vi "CreateTriggerNode.vi"(7 "DOM Document":refnum<k20>, 8 "Error In":errorcluster, 11 "Trigger Configuration":T1={"Input"={"Type"=enum."None", "Timeout (ms)"=1, "Delay (ms)"=0, "Digital IO Line (1-14)"=0, "Digital IO Mode"=enum."Falling"}, "Output"={"Type"=enum."None", "Delay (ms)"=0, "Digital IO Line (1-14)"=1, "Digital IO Mode"=enum."Falling", "Digital IO Pulse Width (sec)"=0.0}} {"Output"."Digital IO Line (1-14)" min=1 max=14 step=1}) -> (0 "Error Out":errorcluster, 3 "Trigger Node":refnum<k20>)   [LabVIEW 2012]
uses:
  TriggerConfiguration.ctl
  TriggerInputConfiguration.ctl
  TriggerInputType.ctl
  driver/Public/Controls/TriggerMode.ctl
  TriggerOutputConfiguration.ctl
  TriggerOutputType.ctl
  libs/LV-Utilities/LV-Utilities.lvlib
  driver/Keithley-2602.lvlib
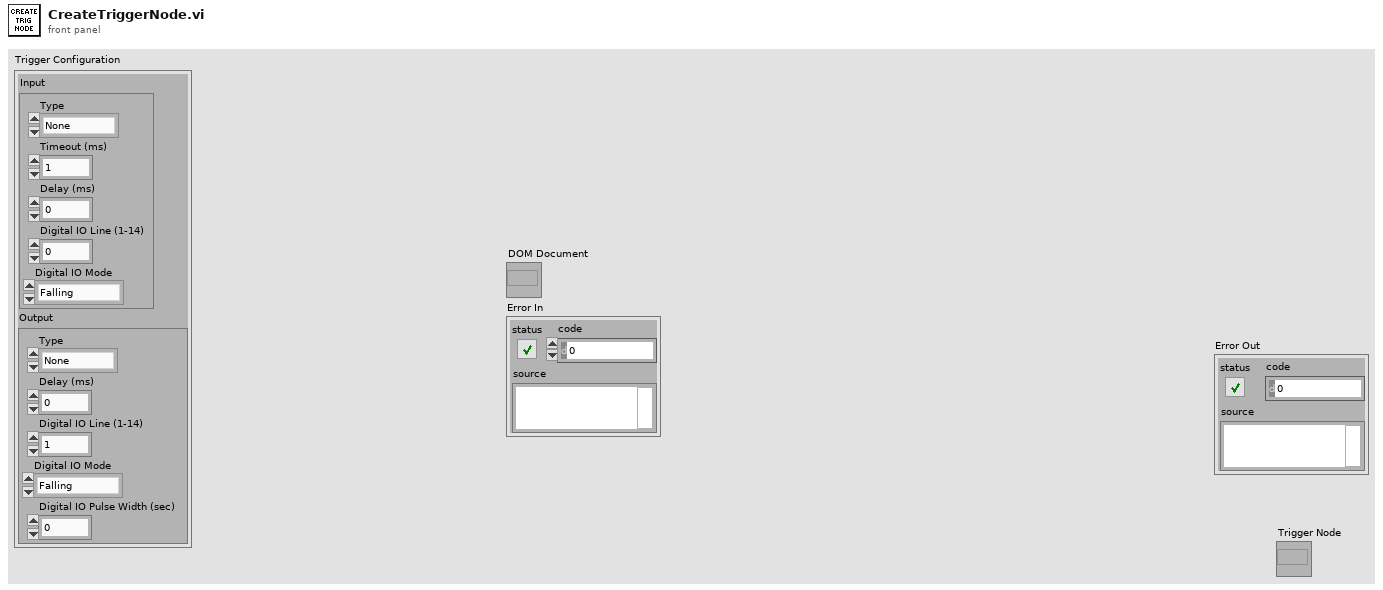
[diagram p1: front panel]
types:
  T1 = typedef "TriggerConfiguration.ctl" = cluster{"Input":T2, "Output":T5}
  T2 = typedef "TriggerInputConfiguration.ctl" = cluster{"Type":T3, "Timeout (ms)":u32, "Delay (ms)":u32, "Digital IO Line (1-14)":u8, "Digital IO Mode":T4}
  T3 = typedef "TriggerInputType.ctl" = enum16{"None", "Digital IO", "Bus"}
  T4 = typedef "Keithley-2602.lvlib/TriggerMode.ctl" = enum16{"Falling", "Rising", "Either", "Synchronous"}
  T5 = typedef "TriggerOutputConfiguration.ctl" = cluster{"Type":T6, "Delay (ms)":u32, "Digital IO Line (1-14)":u8, "Digital IO Mode":T4, "Digital IO Pulse Width (sec)":dbl}
  T6 = typedef "TriggerOutputType.ctl" = enum16{"None", "Digital IO", "Bus"}
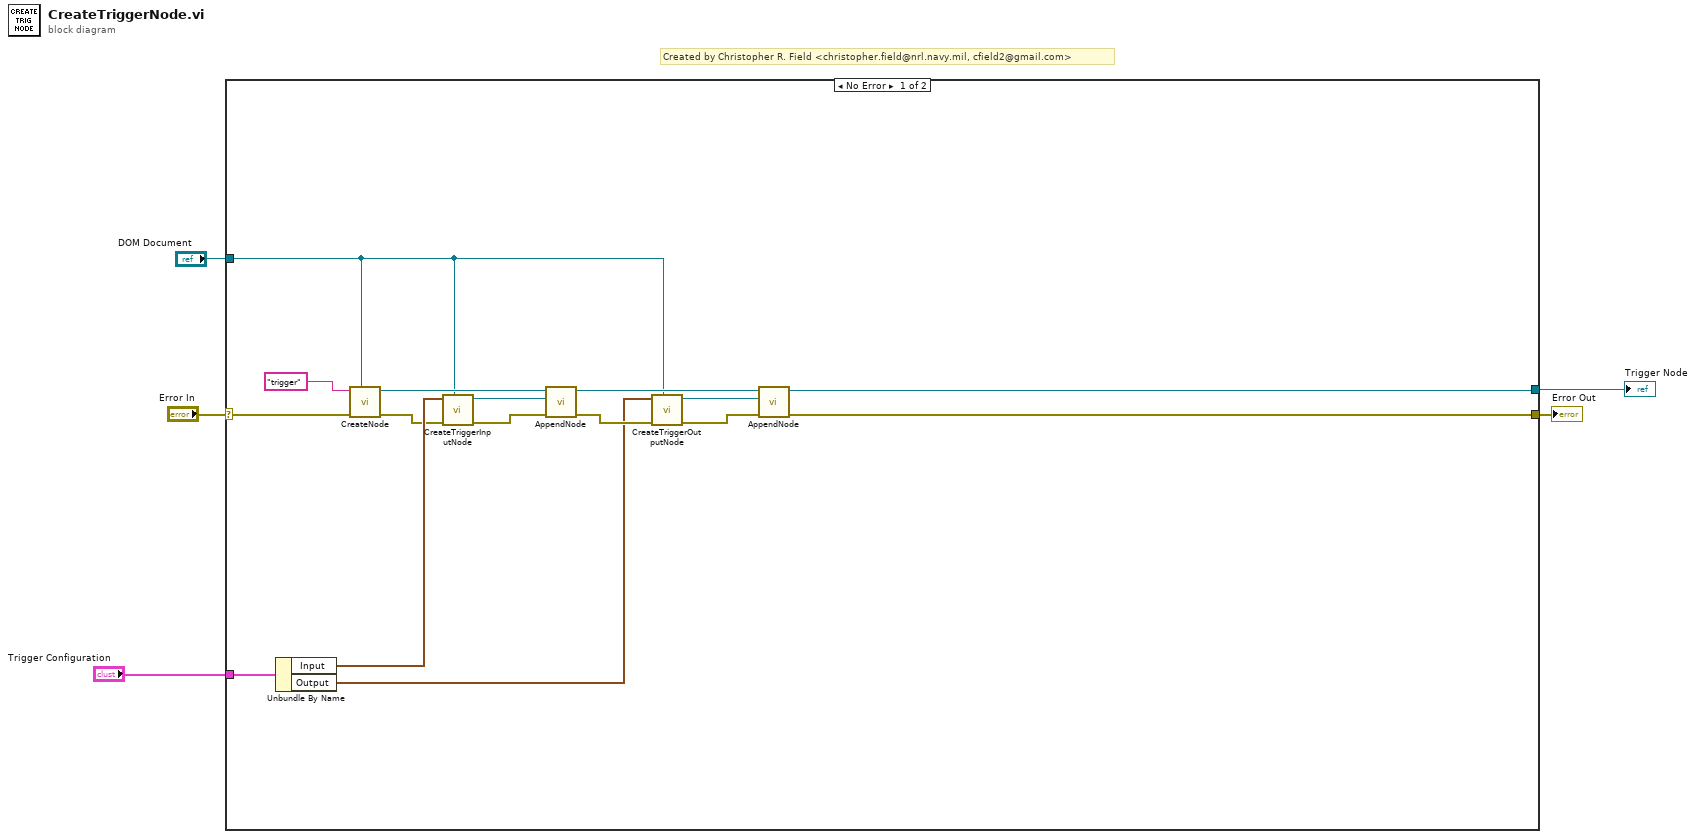
[diagram p0: block diagram]
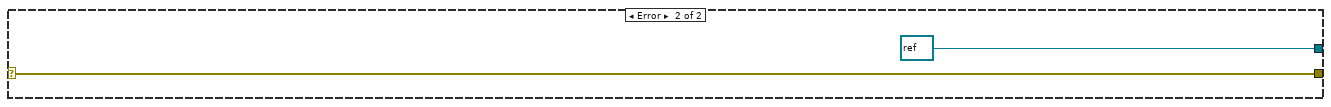
[diagram p2: hidden frame]
diagram:
  # "Created by Christopher R. Field <christopher.field@nrl.navy.mil, cfield2@gmail.com>"
  n1 = case shown="No Error" "Error In" {
    selector: "Error In" -> [w21 w23]
    tunnel: "DOM Document" -> [w9 _]
    tunnel: [w11 w23] -> w3
    tunnel: [w12 refnum<k20> refnum ("DUT Node 2")] -> w2
    tunnel: "Trigger Configuration" -> [w17 _]
    frame No Error {
      n2 = Unbundle By Name(w17) -> ("Input"=w16:T2, "Output"=w8:T5)
      n3 = call "CreateNode.vi"("DOM Document"=w9, "Error In"=w21, "Tag Name"="trigger") -> ("Error out"=w15:errorcluster, "Node"=w19:refnum<k20>)  [unwired: 7 in]
      n4 = call "CreateTriggerInputNode.vi"("DOM Document"=w9, "Error In"=w15, "Trigger Input Configuration"=w16) -> ("Error Out"=w13:errorcluster, "Trigger Input Node"=w14:refnum<k20>)  [unwired: 7 in]
      n5 = call "AppendNode.vi"("Error In"=w13, "Child Node"=w14, "Parent Node In"=w19) -> ("Error Out"=w10:errorcluster, "Parent Node Out"=w18:refnum<k20>)  [unwired: 7 in]
      n6 = call "CreateTriggerOutputNode.vi"("DOM Document"=w9, "Error In"=w10, "Trigger Output Configuration"=w8) -> ("Error Out"=w7:errorcluster, "Trigger Output Node"=w6:refnum<k20>)  [unwired: 7 in]
      n7 = call "AppendNode.vi"("Error In"=w7, "Child Node"=w6, "Parent Node In"=w18) -> ("Error Out"=w11:errorcluster, "Parent Node Out"=w12:refnum<k20>)  [unwired: 7 in]
    }
    frame Error {
    }
  }
  "Error Out" <- w3
  "Trigger Node" <- w2
